vi "SP Convert Filter Cluster.vi"(5 "Conversion":enum16{"Cluster - HTML", "HTML - Cluster"}(ring), 7 "Filter Key Array In":T13, 8 "Filter Cluster In":T1[](array[typedef]) {"Parameter"."Stimulus Port" min=1 step=1; "Parameter"."Response Port" min=1 step=1; "Passband"."Bandwidth Attn" format="%.3g"; "Passband"."Stop/Span" format="%.3g"; "Passband"."Start/Center" format="%.3g"}) -> (1 "Filter Cluster Out":T1[](array[typedef]) {"Parameter"."Stimulus Port" min=1 step=1; "Parameter"."Response Port" min=1 step=1; "Passband"."Bandwidth Attn" format="%.3g"; "Passband"."Stop/Span" format="%.3g"; "Passband"."Start/Center" format="%.3g"}, 2 "Filter HTML Out":string)   [LabVIEW 2011]
uses:
  Addons/internet/utils/keyedarr.llb/Keyed Array.ctl
  TypeDefs/SP Filter.ctl
  TypeDefs/SP Parameter.ctl
  TypeDefs/SP Format.ctl
  TypeDefs/SP Filter Type.ctl
  TypeDefs/SP Filter Passband.ctl
  TypeDefs/SP Frequency Units.ctl
  TypeDefs/SP Frequency Format.ctl
  TypeDefs/SP Filter Ripple.ctl
  TypeDefs/SP Attenuation Point.ctl
  TypeDefs/SP Attenuation Type.ctl
  TypeDefs/SP Skirt Rejection Point.ctl
  TypeDefs/SP Relative Loss.ctl
  Addons/internet/utils/strutil.llb/Case Matching.ctl
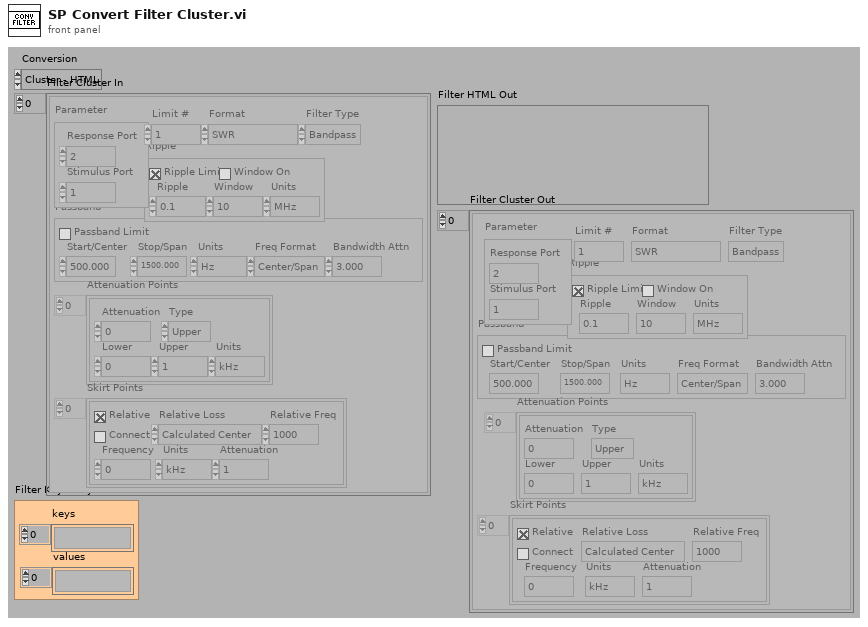
[diagram p1: front panel]
types:
  T1 = typedef "SP Filter.ctl" = cluster{"Limit #":i8, "Parameter":T2, "Format":T3, "Filter Type":T4, "Passband":T5, "Ripple":T8, "Attenuation Points":T9[], "Skirt Points":T11[]}
  T2 = typedef "SP Parameter.ctl" = cluster{"Stimulus Port":i8, "Response Port":i8}
  T3 = typedef "SP Format.ctl" = enum16{"Log Mag", "Lin Mag", "SWR", "Phase", "Expanded Phase", "Delay", "Insertion Loss", "Isolation", "Return Loss"}
  T4 = typedef "SP Filter Type.ctl" = enum16{"Lowpass", "Highpass", "Bandpass", "Bandstop"}
  T5 = typedef "SP Filter Passband.ctl" = cluster{"Start/Center":dbl, "Stop/Span":dbl, "Units":T6, "Freq Format":T7, "Bandwidth Attn":dbl, "Passband Limit":bool}
  T6 = typedef "SP Frequency Units.ctl" = enum16{"Hz", "kHz", "MHz", "GHz", "Points"}
  T7 = typedef "SP Frequency Format.ctl" = enum16{"Start/Stop", "Center/Span"}
  T8 = typedef "SP Filter Ripple.ctl" = cluster{"Ripple Limit":bool, "Window On":bool, "Ripple":dbl, "Window":dbl, "Units":T6}
  T9 = typedef "SP Attenuation Point.ctl" = cluster{"Attenuation":dbl, "Type":T10, "Lower":dbl, "Upper":dbl, "Units":T6}
  T10 = typedef "SP Attenuation Type.ctl" = enum16{"Center", "Lower", "Upper"}
  T11 = typedef "SP Skirt Rejection Point.ctl" = cluster{"Relative":bool, "Connect":bool, "Frequency":dbl, "Units":T6, "Attenuation":dbl, "Relative Loss":T12, "Relative Freq":dbl}
  T12 = typedef "SP Relative Loss.ctl" = enum16{"Calculated Center", "Passband Minimum", "Passband Maximum", "Passband Average", "Frequency"}
  T13 = typedef "Keyed Array.ctl" = cluster{"keys":string[], "values":string[]}
  T14 = typedef "Case Matching.ctl" = enum16{"a != A", "a == A", "system"}
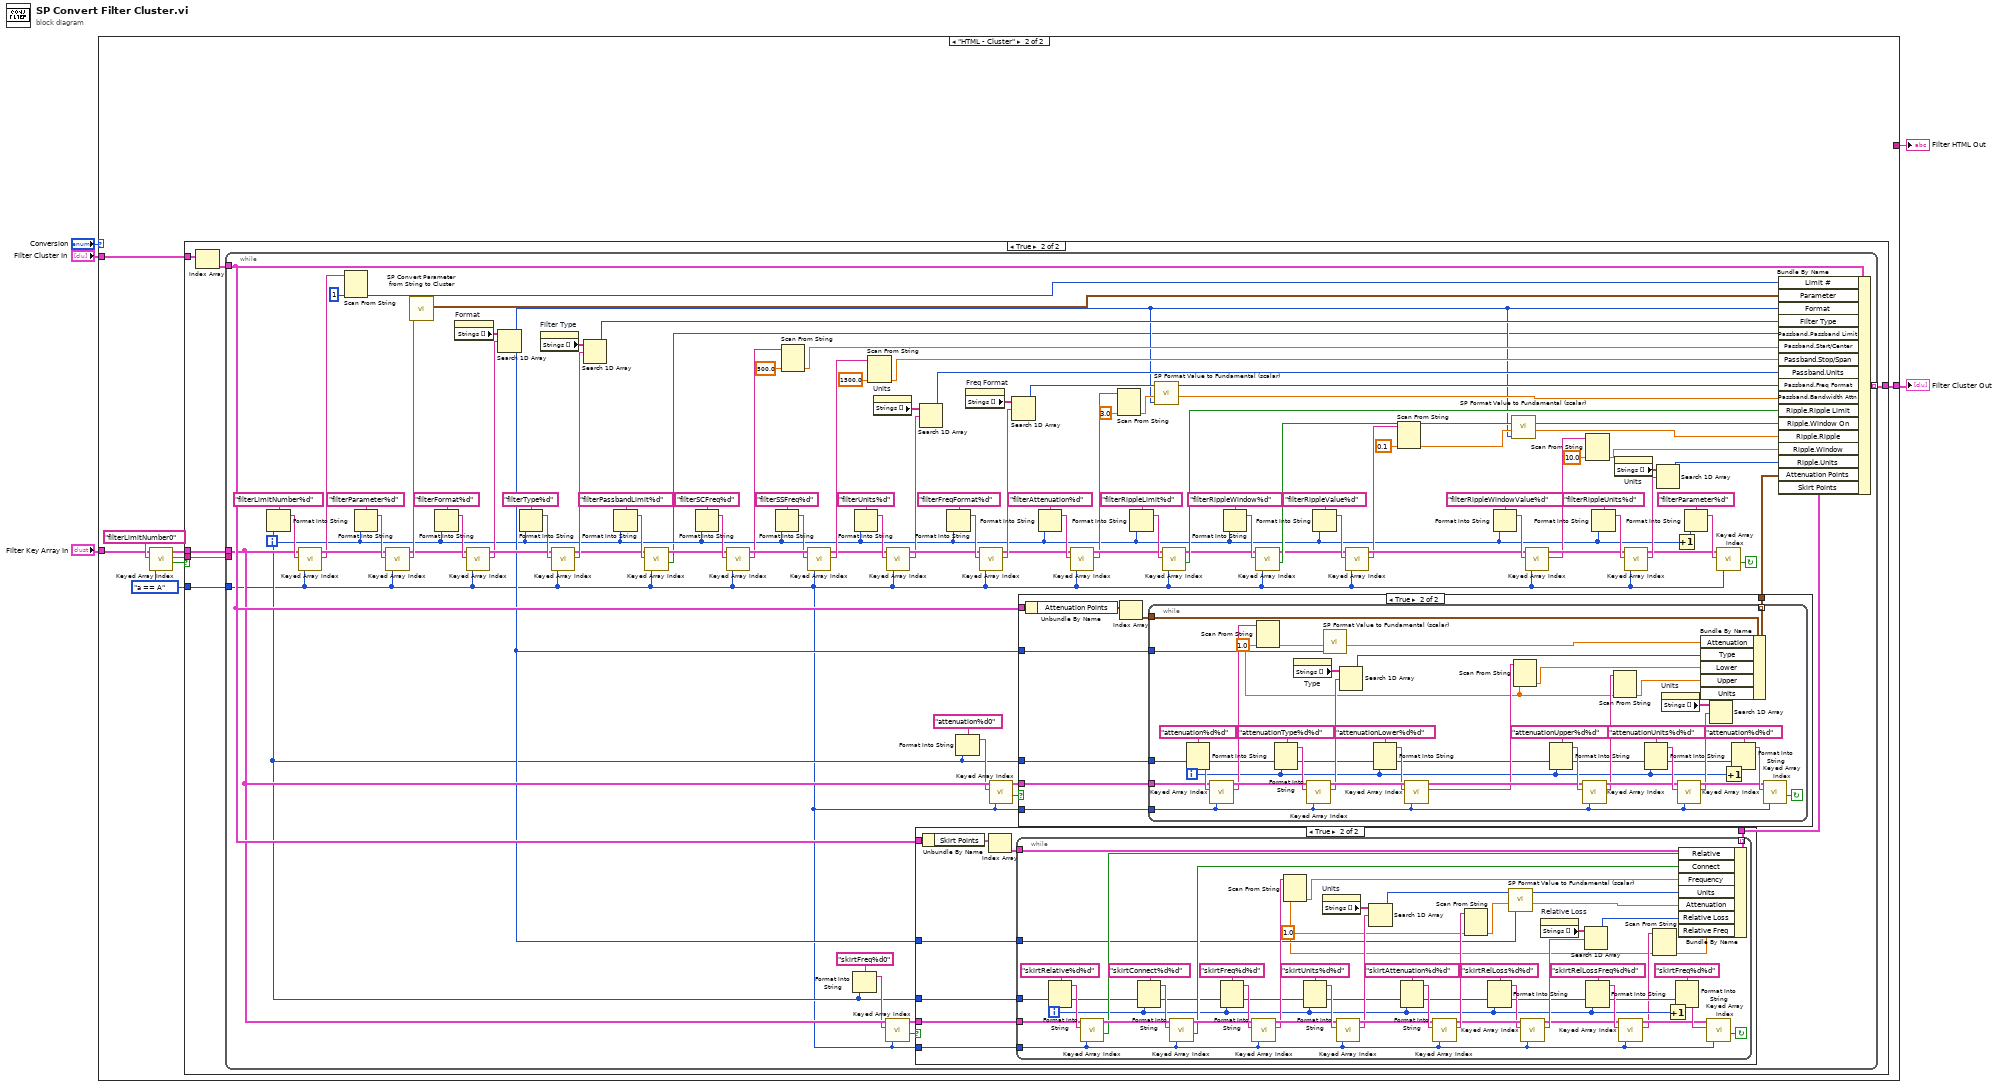
[diagram p0: block diagram]
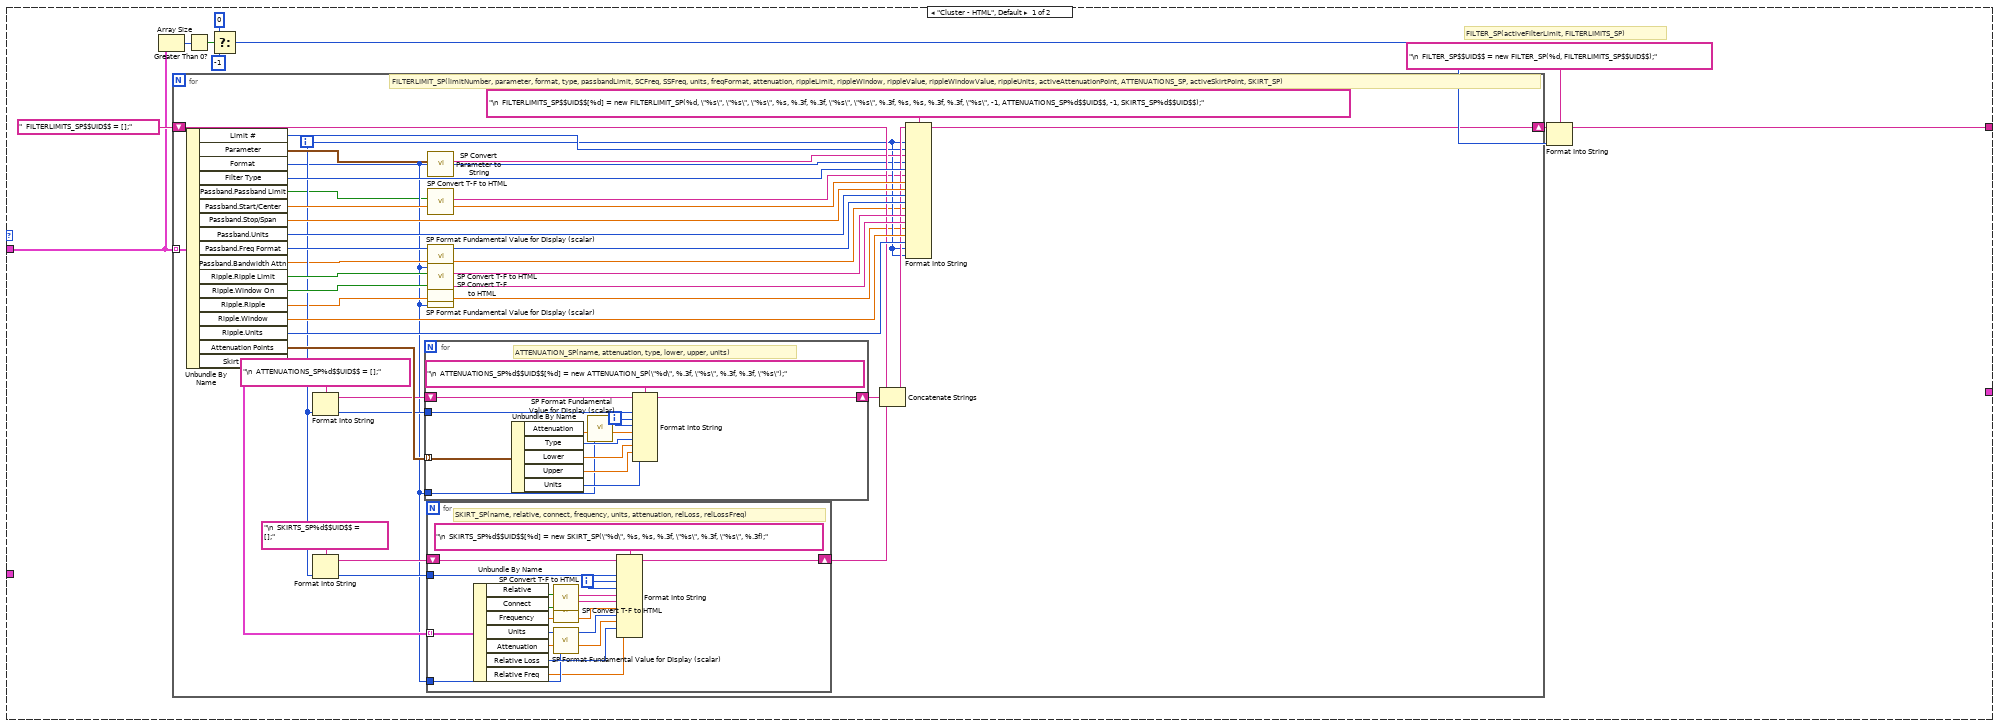
[diagram p2: hidden frame]
diagram:
  n1 = case shown="\"HTML - Cluster\"" "Conversion" {
    tunnel: "Filter Cluster In" -> [w11 w82]
    tunnel: "Filter Key Array In" -> [_ w85]
    tunnel: [w13 _] -> w2
    tunnel: [_ w88] -> w1
    frame "Cluster - HTML", Default {
      # "FILTER_SP(activeFilterLimit, FILTERLIMITS_SP)"
      n2 = Array Size(array=w11) -> (size(s)=w10:i32)
      n3 = for {
        tunnel: w11 -> [w38] mode=indexing
        shift-right: [w31] -> w14
        shift-left: "  FILTERLIMITS_SP$$UID$$ = [];" ("format string") -> [w30]
        i -> [w23]
        # "FILTERLIMIT_SP(limitNumber, parameter, format, type, passbandLimit, SCFreq, SSFreq, units, freqFormat, attenuation, rippleLimit, rippleWindow, rippleValue, rippleWindowValue, rippleUnits, activeAttenuationPoint, ATTENUATIONS_SP, activeSkirtPoint, SKIRT_SP)"
        n4 = Unbundle By Name(w38) -> ("Limit #"=w29:i8, "Parameter"=w36:T2, "Format"=w18:T3, "Filter Type"=w49:T4, "Passband.Passband Limit"=w17:bool, "Passband.Start/Center"=w48:dbl, "Passband.Stop/Span"=w47:dbl, "Passband.Units"=w46:T6, "Passband.Freq Format"=w45:T7, "Passband.Bandwidth Attn"=w22:dbl, "Ripple.Ripple Limit"=w44:bool, "Ripple.Window On"=w43:bool, "Ripple.Ripple"=w20:dbl, "Ripple.Window"=w40:dbl, "Ripple.Units"=w39:T6, "Attenuation Points"=w37:T9[], "Skirt Points"=w32:T11[])
        n5 = Format Into String(format string="\n  ATTENUATIONS_SP%d$$UID$$ = [];", w23) -> (resulting string=w26:string)  [unwired: 2 in, 1 out]
        n6 = Format Into String(format string="\n  SKIRTS_SP%d$$UID$$ = [];", w23) -> (resulting string=w24:string)  [unwired: 2 in, 1 out]
        n7 = for {
          tunnel: w37 -> [w80] mode=indexing
          shift-right: [w77] -> w35
          shift-left: w26 -> [w76]
          tunnel: w23 -> [w71]
          tunnel: w18 -> [w68]
          i -> [w75]
          # "ATTENUATION_SP(name, attenuation, type, lower, upper, units)"
          n8 = Unbundle By Name(w80) -> ("Attenuation"=w70:dbl, "Type"=w78:T10, "Lower"=w74:dbl, "Upper"=w73:dbl, "Units"=w72:T6)
          n9 = call "SP Format Fundamental Value for Display (scalar).vi"("Format"=w68, "Stored Value (0, linear)"=w70) -> ("Display Value"=w69:dbl)  [unwired: 5 out]
          n10 = Format Into String(format string="\n  ATTENUATIONS_SP%d$$UID$$[%d] = new ATTENUATION_SP(\"%d\", %.3f, \"%s\", %.3f, %.3f, \"%s\");", initial string=w76, w71, w75, w75, w69, w78, w74, w73, w72) -> (resulting string=w77:string)  [unwired: 1 in, 1 out]
        }
        n11 = for {
          tunnel: w32 -> [w67] mode=indexing
          shift-right: [w65] -> w34
          shift-left: w24 -> [w64]
          tunnel: w23 -> [w55]
          tunnel: w18 -> [w52]
          i -> [w63]
          # "SKIRT_SP(name, relative, connect, frequency, units, attenuation, relLoss, relLossFreq)"
          n12 = Unbundle By Name(w67) -> ("Relative"=w58:bool, "Connect"=w59:bool, "Frequency"=w62:dbl, "Units"=w61:T6, "Attenuation"=w54:dbl, "Relative Loss"=w60:T12, "Relative Freq"=w51:dbl)
          n13 = call "SP Convert T-F to HTML.vi"("(T/F)"=w58) -> ("HTML (true/false)"=w57:string)  [unwired: 10 out]
          n14 = call "SP Convert T-F to HTML.vi"("(T/F)"=w59) -> ("HTML (true/false)"=w56:string)  [unwired: 10 out]
          n15 = call "SP Format Fundamental Value for Display (scalar).vi"("Format"=w52, "Stored Value (0, linear)"=w54) -> ("Display Value"=w53:dbl)  [unwired: 5 out]
          n16 = Format Into String(format string="\n  SKIRTS_SP%d$$UID$$[%d] = new SKIRT_SP(\"%d\", %s, %s, %.3f, \"%s\", %.3f, \"%s\", %.3f);", initial string=w64, w55, w63, w63, w57, w56, w62, w61, w53, w60, w51) -> (resulting string=w65:string)  [unwired: 1 in, 1 out]
        }
        n17 = call "SP Convert Parameter to String.vi"("Parameter"=w36) -> ("Parameter String"=w28:string)  [unwired: 10 out]
        n18 = call "SP Convert T-F to HTML.vi"("(T/F)"=w17) -> ("HTML (true/false)"=w16:string)  [unwired: 10 out]
        n19 = call "SP Format Fundamental Value for Display (scalar).vi"("Format"=w18, "Stored Value (0, linear)"=w22) -> ("Display Value"=w21:dbl)  [unwired: 5 out]
        n20 = call "SP Convert T-F to HTML.vi"("(T/F)"=w44) -> ("HTML (true/false)"=w42:string)  [unwired: 10 out]
        n21 = call "SP Convert T-F to HTML.vi"("(T/F)"=w43) -> ("HTML (true/false)"=w41:string)  [unwired: 10 out]
        n22 = call "SP Format Fundamental Value for Display (scalar).vi"("Format"=w18, "Stored Value (0, linear)"=w20) -> ("Display Value"=w19:dbl)  [unwired: 5 out]
        n23 = Concatenate Strings(w30, w35, w34) -> (w33:string)
        n24 = Format Into String(format string="\n  FILTERLIMITS_SP$$UID$$[%d] = new FILTERLIMIT_SP(%d, \"%s\", \"%s\", \"%s\", %s, %.3f, %.3f, \"%s\", \"%s\", %.3f, %s, %s, %.3f, %.3f, \"%s\", -1, ATTENUATIONS_SP%d$$UID$$, -1, SKIRTS_SP%d$$UID$$);", initial string=w33, w23, w29, w28, w18, w49, w16, w48, w47, w46, w45, w21, w42, w41, w19, w40, w39, w23, w23) -> (resulting string=w31:string)  [unwired: 1 in, 1 out]
      }
      n25 = Greater Than 0?(x=w10) -> (x > 0?=w9:bool)
      n26 = Select(t=i8 0, s=w9, f=i8 -1) -> (s? t:f=w6:i8)
      n27 = Format Into String(format string="\n  FILTER_SP$$UID$$ = new FILTER_SP(%d, FILTERLIMITS_SP$$UID$$);", initial string=w14, w6) -> (resulting string=w13:string)  [unwired: 1 in, 1 out]
    }
    frame "HTML - Cluster" {
      w81 = Case_Matching."a == A" ("case matching (sensitive)")
      n28 = call "Keyed Array Index.vi"("case matching (sensitive)"=w81, "key"="filterLimitNumber0", "array in"=w85) -> ("valid key"=w83:bool, "value"=w86:string, "duplicate array"=w84:T13)  [unwired: 1 in, 1 out]
      n29 = case shown="True" w83 {
        tunnel: [_ w94] -> w88
        tunnel: w86 -> [_ w93]
        tunnel: w84 -> [_ w92]
        tunnel: w82 -> [_ w91]
        tunnel: w81 -> [_ w89]
        frame False {
        }
        frame True {
          n30 = Index Array(array=w91) -> (element=w90:T1)  [unwired: 1 in]
          n31 = while {
            tunnel: [w197] -> w94 mode=indexing
            tunnel: w93 -> [_]
            tunnel: w92 -> [w129]
            tunnel: w90 -> [w170]
            tunnel: w89 -> [w96]
            i -> [w99]
            stop <- w136 continue-if-true
            n32 = Format Into String(format string="filterLimitNumber%d", w99) -> (resulting string=w131:string)  [unwired: 2 in, 1 out]
            n33 = call "Keyed Array Index.vi"("case matching (sensitive)"=w96, "key"=w131, "array in"=w129) -> ("value"=w127:string, "duplicate array"=w130:T13)  [unwired: 1 in, 2 out]
            n34 = Scan From String(input string=w127, default 1=i8 1 ("default value 1")) -> (output 1=w126:i8)  [unwired: 3 in, 3 out]
            n35 = Format Into String(format string="filterParameter%d", w99) -> (resulting string=w172:string)  [unwired: 2 in, 1 out]
            n36 = call "Keyed Array Index.vi"("case matching (sensitive)"=w96, "key"=w172, "array in"=w130) -> ("value"=w169:string, "duplicate array"=w123:T13)  [unwired: 1 in, 2 out]
            n37 = call "SP Convert Parameter from String to Cluster.vi"("Parameter String"=w169) -> ("Parameter"=w187:T2)  [unwired: 10 out]
            n38 = Format Into String(format string="filterFormat%d", w99) -> (resulting string=w124:string)  [unwired: 2 in, 1 out]
            n39 = property on="Format" class="Enum (strict)"() -> ("Strings []"=w121:string[])  [unwired: 2 in, 2 out]
            n40 = call "Keyed Array Index.vi"("case matching (sensitive)"=w96, "key"=w124, "array in"=w123) -> ("value"=w120:string, "duplicate array"=w122:T13)  [unwired: 1 in, 2 out]
            n41 = Search 1D Array(1D array=w121, element=w120) -> (index of element=w106:i32)  [unwired: 1 out]
            n42 = Format Into String(format string="filterType%d", w99) -> (resulting string=w175:string)  [unwired: 2 in, 1 out]
            n43 = property on="Filter Type" class="Enum (strict)"() -> ("Strings []"=w133:string[])  [unwired: 2 in, 2 out]
            n44 = call "Keyed Array Index.vi"("case matching (sensitive)"=w96, "key"=w175, "array in"=w122) -> ("value"=w168:string, "duplicate array"=w98:T13)  [unwired: 1 in, 2 out]
            n45 = Search 1D Array(1D array=w133, element=w168) -> (index of element=w198:i32)  [unwired: 1 out]
            n46 = Format Into String(format string="filterPassbandLimit%d", w99) -> (resulting string=w100:string)  [unwired: 2 in, 1 out]
            n47 = call "Keyed Array Index.vi"("case matching (sensitive)"=w96, "key"=w100, "array in"=w98) -> ("valid key"=w95:bool, "duplicate array"=w97:T13)  [unwired: 1 in, 2 out]
            n48 = Format Into String(format string="filterSCFreq%d", w99) -> (resulting string=w176:string)  [unwired: 2 in, 1 out]
            n49 = call "Keyed Array Index.vi"("case matching (sensitive)"=w96, "key"=w176, "array in"=w97) -> ("value"=w167:string, "duplicate array"=w178:T13)  [unwired: 1 in, 2 out]
            n50 = Format Into String(format string="filterSSFreq%d", w99) -> (resulting string=w177:string)  [unwired: 2 in, 1 out]
            n51 = Scan From String(input string=w167, default 1=500.0 ("default value 1")) -> (output 1=w196:dbl)  [unwired: 3 in, 3 out]
            n52 = call "Keyed Array Index.vi"("case matching (sensitive)"=w96, "key"=w177, "array in"=w178) -> ("value"=w166:string, "duplicate array"=w159:T13)  [unwired: 1 in, 2 out]
            n53 = Format Into String(format string="skirtFreq%d0", w99) -> (resulting string=w102:string)  [unwired: 2 in, 1 out]
            n54 = Format Into String(format string="filterUnits%d", w99) -> (resulting string=w165:string)  [unwired: 2 in, 1 out]
            n55 = Scan From String(input string=w166, default 1=1500.0 ("default value 1")) -> (output 1=w195:dbl)  [unwired: 3 in, 3 out]
            n56 = property on="Units" class="Enum (strict)"() -> ("Strings []"=w118:string[])  [unwired: 2 in, 2 out]
            n57 = call "Keyed Array Index.vi"("case matching (sensitive)"=w96, "key"=w102, "array in"=w129) -> ("valid key"=w186:bool, "duplicate array"=w185:T13)  [unwired: 1 in, 2 out]
            n58 = call "Keyed Array Index.vi"("case matching (sensitive)"=w96, "key"=w165, "array in"=w159) -> ("value"=w157:string, "duplicate array"=w158:T13)  [unwired: 1 in, 2 out]
            n59 = case shown="True" w186 {
              tunnel: w170 -> [_ w206]
              tunnel: w185 -> [_ w204]
              tunnel: w96 -> [_ w203]
              tunnel: [_ w202] -> w184
              tunnel: w99 -> [_ w200]
              tunnel: w106 -> [_ w199]
              frame False {
              }
              frame True {
                n60 = Unbundle By Name(w206) -> ("Skirt Points"=w201:T11[])
                n61 = Index Array(array=w201) -> (element=w205:T11)  [unwired: 1 in]
                n62 = while {
                  tunnel: w205 -> [w252]
                  tunnel: w203 -> [w208]
                  tunnel: w204 -> [w242]
                  tunnel: [w235] -> w202 mode=indexing
                  tunnel: w200 -> [w214]
                  tunnel: w199 -> [w217]
                  i -> [w213]
                  stop <- w243 continue-if-true
                  w207 = 1.0 ("default value 1")
                  n63 = Format Into String(format string="skirtRelative%d%d", w214, w213) -> (resulting string=w250:string)  [unwired: 2 in, 1 out]
                  n64 = call "Keyed Array Index.vi"("case matching (sensitive)"=w208, "key"=w250, "array in"=w242) -> ("valid key"=w232:bool, "duplicate array"=w253:T13)  [unwired: 1 in, 2 out]
                  n65 = Format Into String(format string="skirtConnect%d%d", w214, w213) -> (resulting string=w247:string)  [unwired: 2 in, 1 out]
                  n66 = call "Keyed Array Index.vi"("case matching (sensitive)"=w208, "key"=w247, "array in"=w253) -> ("valid key"=w231:bool, "duplicate array"=w254:T13)  [unwired: 1 in, 2 out]
                  n67 = Format Into String(format string="skirtFreq%d%d", w214, w213) -> (resulting string=w246:string)  [unwired: 2 in, 1 out]
                  n68 = call "Keyed Array Index.vi"("case matching (sensitive)"=w208, "key"=w246, "array in"=w254) -> ("value"=w234:string, "duplicate array"=w238:T13)  [unwired: 1 in, 2 out]
                  n69 = Scan From String(input string=w234, default 1=w207) -> (output 1=w233:dbl)  [unwired: 3 in, 3 out]
                  n70 = Format Into String(format string="skirtUnits%d%d", w214, w213) -> (resulting string=w239:string)  [unwired: 2 in, 1 out]
                  n71 = property on="Units" class="Enum (strict)"() -> ("Strings []"=w221:string[])  [unwired: 2 in, 2 out]
                  n72 = call "Keyed Array Index.vi"("case matching (sensitive)"=w208, "key"=w239, "array in"=w238) -> ("value"=w230:string, "duplicate array"=w237:T13)  [unwired: 1 in, 2 out]
                  n73 = Search 1D Array(1D array=w221, element=w230) -> (index of element=w223:i32)  [unwired: 1 out]
                  n74 = Format Into String(format string="skirtAttenuation%d%d", w214, w213) -> (resulting string=w240:string)  [unwired: 2 in, 1 out]
                  n75 = call "Keyed Array Index.vi"("case matching (sensitive)"=w208, "key"=w240, "array in"=w237) -> ("value"=w229:string, "duplicate array"=w227:T13)  [unwired: 1 in, 2 out]
                  n76 = Scan From String(input string=w229, default 1=w207) -> (output 1=w219:dbl)  [unwired: 3 in, 3 out]
                  n77 = Format Into String(format string="skirtRelLoss%d%d", w214, w213) -> (resulting string=w226:string)  [unwired: 2 in, 1 out]
                  n78 = call "SP Format Value to Fundamental (scalar).vi"("Display Format"=w217, "Displayed Value (0)"=w219) -> ("Stored Value"=w218:dbl)  [unwired: 5 out]
                  n79 = call "Keyed Array Index.vi"("case matching (sensitive)"=w208, "key"=w226, "array in"=w227) -> ("value"=w224:string, "duplicate array"=w212:T13)  [unwired: 1 in, 2 out]
                  n80 = property on="Relative Loss" class="Enum (strict)"() -> ("Strings []"=w220:string[])  [unwired: 2 in, 2 out]
                  n81 = Search 1D Array(1D array=w220, element=w224) -> (index of element=w225:i32)  [unwired: 1 out]
                  n82 = Format Into String(format string="skirtRelLossFreq%d%d", w214, w213) -> (resulting string=w216:string)  [unwired: 2 in, 1 out]
                  n83 = call "Keyed Array Index.vi"("case matching (sensitive)"=w208, "key"=w216, "array in"=w212) -> ("value"=w210:string, "duplicate array"=w211:T13)  [unwired: 1 in, 2 out]
                  n84 = Scan From String(input string=w210, default 1=w207) -> (output 1=w209:dbl)  [unwired: 3 in, 3 out]
                  n85 = Increment(x=w213) -> (x+1=w222:i32)
                  n86 = Format Into String(format string="skirtFreq%d%d", w214, w222) -> (resulting string=w244:string)  [unwired: 2 in, 1 out]
                  n87 = Bundle By Name(cluster=w252, "Relative"=w232, "Connect"=w231, "Frequency"=w233, "Units"=w223, "Attenuation"=w218, "Relative Loss"=w225, "Relative Freq"=w209) -> (w235:T11)
                  n88 = call "Keyed Array Index.vi"("case matching (sensitive)"=w208, "key"=w244, "array in"=w211) -> ("valid key"=w243:bool)  [unwired: 1 in, 3 out]
                }
              }
            }
            n89 = Search 1D Array(1D array=w118, element=w157) -> (index of element=w194:i32)  [unwired: 1 out]
            n90 = Format Into String(format string="filterFreqFormat%d", w99) -> (resulting string=w162:string)  [unwired: 2 in, 1 out]
            n91 = Format Into String(format string="attenuation%d0", w99) -> (resulting string=w104:string)  [unwired: 2 in, 1 out]
            n92 = property on="Freq Format" class="Enum (strict)"() -> ("Strings []"=w119:string[])  [unwired: 2 in, 2 out]
            n93 = call "Keyed Array Index.vi"("case matching (sensitive)"=w96, "key"=w162, "array in"=w158) -> ("value"=w156:string, "duplicate array"=w112:T13)  [unwired: 1 in, 2 out]
            n94 = call "Keyed Array Index.vi"("case matching (sensitive)"=w96, "key"=w104, "array in"=w129) -> ("valid key"=w189:bool, "duplicate array"=w190:T13)  [unwired: 1 in, 2 out]
            n95 = Search 1D Array(1D array=w119, element=w156) -> (index of element=w193:i32)  [unwired: 1 out]
            n96 = case shown="True" w189 {
              tunnel: w170 -> [_ w262]
              tunnel: w190 -> [_ w259]
              tunnel: w96 -> [_ w258]
              tunnel: [_ w257] -> w188
              tunnel: w99 -> [_ w256]
              tunnel: w106 -> [_ w255]
              frame False {
              }
              frame True {
                n97 = Unbundle By Name(w262) -> ("Attenuation Points"=w260:T9[])
                n98 = Index Array(array=w260) -> (element=w261:T9)  [unwired: 1 in]
                n99 = while {
                  tunnel: w261 -> [w271]
                  tunnel: w258 -> [w284]
                  tunnel: w259 -> [w290]
                  tunnel: [w282] -> w257 mode=indexing
                  tunnel: w256 -> [w269]
                  tunnel: w255 -> [w263]
                  i -> [w268]
                  stop <- w291 continue-if-true
                  w277 = 1.0 ("default value 1")
                  n100 = Format Into String(format string="attenuation%d%d", w269, w268) -> (resulting string=w299:string)  [unwired: 2 in, 1 out]
                  n101 = call "Keyed Array Index.vi"("case matching (sensitive)"=w284, "key"=w299, "array in"=w290) -> ("value"=w298:string, "duplicate array"=w301:T13)  [unwired: 1 in, 2 out]
                  n102 = Scan From String(input string=w298, default 1=w277) -> (output 1=w265:dbl)  [unwired: 3 in, 3 out]
                  n103 = Format Into String(format string="attenuationType%d%d", w269, w268) -> (resulting string=w295:string)  [unwired: 2 in, 1 out]
                  n104 = property on="Type" class="Enum (strict)"() -> ("Strings []"=w266:string[])  [unwired: 2 in, 2 out]
                  n105 = call "Keyed Array Index.vi"("case matching (sensitive)"=w284, "key"=w295, "array in"=w301) -> ("value"=w278:string, "duplicate array"=w302:T13)  [unwired: 1 in, 2 out]
                  n106 = call "SP Format Value to Fundamental (scalar).vi"("Display Format"=w263, "Displayed Value (0)"=w265) -> ("Stored Value"=w264:dbl)  [unwired: 5 out]
                  n107 = Search 1D Array(1D array=w266, element=w278) -> (index of element=w272:i32)  [unwired: 1 out]
                  n108 = Format Into String(format string="attenuationLower%d%d", w269, w268) -> (resulting string=w294:string)  [unwired: 2 in, 1 out]
                  n109 = call "Keyed Array Index.vi"("case matching (sensitive)"=w284, "key"=w294, "array in"=w302) -> ("value"=w281:string, "duplicate array"=w286:T13)  [unwired: 1 in, 2 out]
                  n110 = Scan From String(input string=w281, default 1=w277) -> (output 1=w273:dbl)  [unwired: 3 in, 3 out]
                  n111 = Format Into String(format string="attenuationUpper%d%d", w269, w268) -> (resulting string=w287:string)  [unwired: 2 in, 1 out]
                  n112 = call "Keyed Array Index.vi"("case matching (sensitive)"=w284, "key"=w287, "array in"=w286) -> ("value"=w280:string, "duplicate array"=w285:T13)  [unwired: 1 in, 2 out]
                  n113 = Scan From String(input string=w280, default 1=w277) -> (output 1=w274:dbl)  [unwired: 3 in, 3 out]
                  n114 = Format Into String(format string="attenuationUnits%d%d", w269, w268) -> (resulting string=w288:string)  [unwired: 2 in, 1 out]
                  n115 = property on="Units" class="Enum (strict)"() -> ("Strings []"=w267:string[])  [unwired: 2 in, 2 out]
                  n116 = call "Keyed Array Index.vi"("case matching (sensitive)"=w284, "key"=w288, "array in"=w285) -> ("value"=w276:string, "duplicate array"=w279:T13)  [unwired: 1 in, 2 out]
                  n117 = Search 1D Array(1D array=w267, element=w276) -> (index of element=w275:i32)  [unwired: 1 out]
                  n118 = Bundle By Name(cluster=w271, "Attenuation"=w264, "Type"=w272, "Lower"=w273, "Upper"=w274, "Units"=w275) -> (w282:T9)
                  n119 = Increment(x=w268) -> (x+1=w270:i32)
                  n120 = Format Into String(format string="attenuation%d%d", w269, w270) -> (resulting string=w292:string)  [unwired: 2 in, 1 out]
                  n121 = call "Keyed Array Index.vi"("case matching (sensitive)"=w284, "key"=w292, "array in"=w279) -> ("valid key"=w291:bool)  [unwired: 1 in, 3 out]
                }
              }
            }
            n122 = Format Into String(format string="filterAttenuation%d", w99) -> (resulting string=w113:string)  [unwired: 2 in, 1 out]
            n123 = call "Keyed Array Index.vi"("case matching (sensitive)"=w96, "key"=w113, "array in"=w112) -> ("value"=w109:string, "duplicate array"=w111:T13)  [unwired: 1 in, 2 out]
            n124 = Scan From String(input string=w109, default 1=3.0 ("default value 1")) -> (output 1=w108:dbl)  [unwired: 3 in, 3 out]
            n125 = Format Into String(format string="filterRippleLimit%d", w99) -> (resulting string=w161:string)  [unwired: 2 in, 1 out]
            n126 = call "SP Format Value to Fundamental (scalar).vi"("Display Format"=w106, "Displayed Value (0)"=w108) -> ("Stored Value"=w107:dbl)  [unwired: 5 out]
            n127 = call "Keyed Array Index.vi"("case matching (sensitive)"=w96, "key"=w161, "array in"=w111) -> ("valid key"=w149:bool, "duplicate array"=w147:T13)  [unwired: 1 in, 2 out]
            n128 = Format Into String(format string="filterRippleWindow%d", w99) -> (resulting string=w154:string)  [unwired: 2 in, 1 out]
            n129 = call "Keyed Array Index.vi"("case matching (sensitive)"=w96, "key"=w154, "array in"=w147) -> ("valid key"=w148:bool, "duplicate array"=w146:T13)  [unwired: 1 in, 2 out]
            n130 = Format Into String(format string="filterRippleValue%d", w99) -> (resulting string=w153:string)  [unwired: 2 in, 1 out]
            n131 = call "Keyed Array Index.vi"("case matching (sensitive)"=w96, "key"=w153, "array in"=w146) -> ("value"=w134:string, "duplicate array"=w145:T13)  [unwired: 1 in, 2 out]
            n132 = Scan From String(input string=w134, default 1=0.1 ("default value 1")) -> (output 1=w116:dbl)  [unwired: 3 in, 3 out]
            n133 = Format Into String(format string="filterRippleWindowValue%d", w99) -> (resulting string=w150:string)  [unwired: 2 in, 1 out]
            n134 = call "SP Format Value to Fundamental (scalar).vi"("Display Format"=w106, "Displayed Value (0)"=w116) -> ("Stored Value"=w115:dbl)  [unwired: 5 out]
            n135 = call "Keyed Array Index.vi"("case matching (sensitive)"=w96, "key"=w150, "array in"=w145) -> ("value"=w141:string, "duplicate array"=w142:T13)  [unwired: 1 in, 2 out]
            n136 = Scan From String(input string=w141, default 1=10.0 ("default value 1")) -> (output 1=w192:dbl)  [unwired: 3 in, 3 out]
            n137 = Format Into String(format string="filterRippleUnits%d", w99) -> (resulting string=w144:string)  [unwired: 2 in, 1 out]
            n138 = property on="Units" class="Enum (strict)"() -> ("Strings []"=w117:string[])  [unwired: 2 in, 2 out]
            n139 = call "Keyed Array Index.vi"("case matching (sensitive)"=w96, "key"=w144, "array in"=w142) -> ("value"=w140:string, "duplicate array"=w135:T13)  [unwired: 1 in, 2 out]
            n140 = Search 1D Array(1D array=w117, element=w140) -> (index of element=w191:i32)  [unwired: 1 out]
            n141 = Increment(x=w99) -> (x+1=w137:i32)
            n142 = Format Into String(format string="filterParameter%d", w137) -> (resulting string=w138:string)  [unwired: 2 in, 1 out]
            n143 = call "Keyed Array Index.vi"("case matching (sensitive)"=w96, "key"=w138, "array in"=w135) -> ("valid key"=w136:bool)  [unwired: 1 in, 3 out]
            n144 = Bundle By Name(cluster=w170, "Limit #"=w126, "Parameter"=w187, "Format"=w106, "Filter Type"=w198, "Passband.Passband Limit"=w95, "Passband.Start/Center"=w196, "Passband.Stop/Span"=w195, "Passband.Units"=w194, "Passband.Freq Format"=w193, "Passband.Bandwidth Attn"=w107, "Ripple.Ripple Limit"=w149, "Ripple.Window On"=w148, "Ripple.Ripple"=w115, "Ripple.Window"=w192, "Ripple.Units"=w191, "Attenuation Points"=w188, "Skirt Points"=w184) -> (w197:T1)
          }
        }
      }
    }
  }
  "Filter HTML Out" <- w2
  "Filter Cluster Out" <- w1
